vi "Read Group Properties.vi"(11 "Tree path":string) -> ()   [LabVIEW 2017]
uses:
  <vilib>/Utility/error.llb/DialogType.ctl
  Global Data Analysis.vi
  Data Manipulation/Global_Var_CMS_SQC.vi
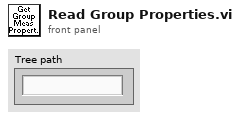
[diagram p1: front panel]
types:
  T1 = typedef "DialogType.ctl" = u16
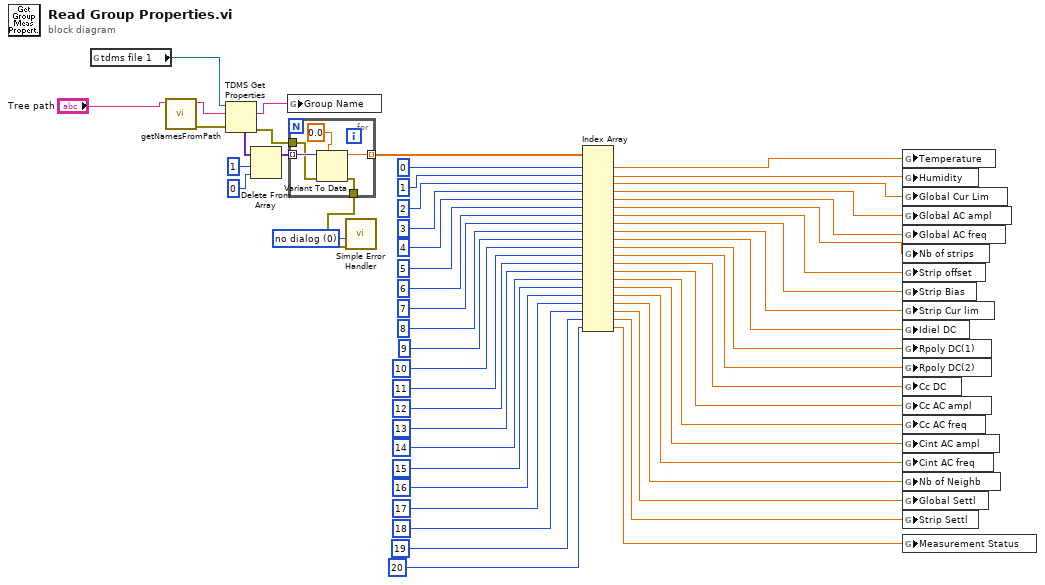
[diagram p0: block diagram]
diagram:
  w8 = T1 0 items=["no dialog", "OK message", "continue or stop message", "OK message + warnings", "continue/stop + warnings"] ("type of dialog (OK msg:1)")
  n1 = global read "Global Data Analysis.vi" "tdms file 1"() -> (w51:refnum<k34>)
  n2 = call <vilib>:"getNamesFromPath.vi"("tree path"="Tree path") -> ("error out"=w11:errorcluster, "group"=w13:string)  [unwired: 1 in, 4 out]
  n3 = TDMS Get Properties(8:w11, 10:w13, 11:w51) -> (0:w10:errorcluster, 2:w1:string, 4:w52:variant[])  [unwired: 1 in, 5 out]
  n4 = Delete From Array(array=w52, length=1, index=0 ("length")) -> (array with subset deleted=w55:variant[])  [unwired: 1 out]
  n5 = global write "Global_Var_CMS_SQC.vi" "Group Name"(w1) -> ()
  n6 = for {
    tunnel: [w60] -> w33 mode=indexing
    tunnel: w55 -> [w59] mode=indexing
    tunnel: [w57] -> w9
    tunnel: w10 -> [w56]
    n7 = Variant To Data(error in=w56, type=0.0, Variant=w59) -> (data=w60:dbl, error out=w57:errorcluster)
  }
  n8 = call <vilib>:"Simple Error Handler.vi"("type of dialog (OK msg:1)"=w8, "error in (no error)"=w9) -> ()  [unwired: 3 in, 5 out]
  n9 = Index Array(array=w33, index #1=0 ("length"), index #2=1 ("index"), index #3=2 ("index"), index #4=3 ("index"), index #5=4 ("index"), index #6=5 ("index"), index #7=6 ("index"), index #8=7 ("index"), index #9=8 ("index"), index #10=9 ("index"), index #11=10 ("index"), index #12=11 ("index"), index #13=12 ("index"), index #14=13 ("index"), index #15=14 ("index"), index #16=15 ("index"), index #17=16 ("index"), index #18=17 ("index"), index #19=18 ("index"), index #20=19 ("index"), index #21=20 ("index")) -> (element #1=w32:dbl, element #2=w31:dbl, element #3=w30:dbl, element #4=w29:dbl, element #5=w28:dbl, element #6=w27:dbl, element #7=w26:dbl, element #8=w25:dbl, element #9=w24:dbl, element #10=w23:dbl, element #11=w22:dbl, element #12=w21:dbl, element #13=w20:dbl, element #14=w19:dbl, element #15=w18:dbl, element #16=w17:dbl, element #17=w16:dbl, element #18=w14:dbl, element #19=w6:dbl, element #20=w5:dbl, element #21=w2:dbl)
  n10 = global write "Global Data Analysis.vi" "Temperature"(w32) -> ()
  n11 = global write "Global Data Analysis.vi" "Humidity"(w31) -> ()
  n12 = global write "Global Data Analysis.vi" "Global Cur Lim"(w30) -> ()
  n13 = global write "Global Data Analysis.vi" "Global AC ampl"(w29) -> ()
  n14 = global write "Global Data Analysis.vi" "Global AC freq"(w28) -> ()
  n15 = global write "Global Data Analysis.vi" "Nb of strips"(w27) -> ()
  n16 = global write "Global Data Analysis.vi" "Strip offset"(w26) -> ()
  n17 = global write "Global Data Analysis.vi" "Strip Bias"(w25) -> ()
  n18 = global write "Global Data Analysis.vi" "Strip Cur lim"(w24) -> ()
  n19 = global write "Global Data Analysis.vi" "Idiel DC"(w23) -> ()
  n20 = global write "Global Data Analysis.vi" "Rpoly DC(1)"(w22) -> ()
  n21 = global write "Global Data Analysis.vi" "Rpoly DC(2)"(w21) -> ()
  n22 = global write "Global Data Analysis.vi" "Cc DC"(w20) -> ()
  n23 = global write "Global Data Analysis.vi" "Cc AC ampl"(w19) -> ()
  n24 = global write "Global Data Analysis.vi" "Cc AC freq"(w18) -> ()
  n25 = global write "Global Data Analysis.vi" "Cint AC ampl"(w17) -> ()
  n26 = global write "Global Data Analysis.vi" "Cint AC freq"(w16) -> ()
  n27 = global write "Global Data Analysis.vi" "Nb of Neighb"(w14) -> ()
  n28 = global write "Global Data Analysis.vi" "Global Settl"(w6) -> ()
  n29 = global write "Global Data Analysis.vi" "Strip Settl"(w5) -> ()
  n30 = global write "Global Data Analysis.vi" "Measurement Status"(w2) -> ()
